vi "PlotFramePositions.vi"() -> ()   [LabVIEW 2012]
panel:
  in  "Frame Size":i16[](array[numeric])
  in  "Coordinates out":dbl[][](array[numeric])
  out "2D Picture":picture
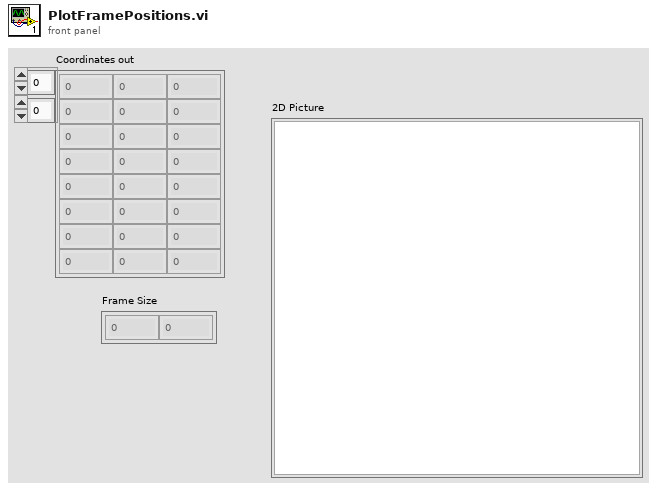
[diagram p1: front panel]
types:
  T1 = cluster{"Width":i16, "Style":enum32{"Solid", "Dash", "Dot", "DashDot", "DashDotDot"}}
  T2 = cluster{"left":i16, "top":i16, "right":i16, "bottom":i16}
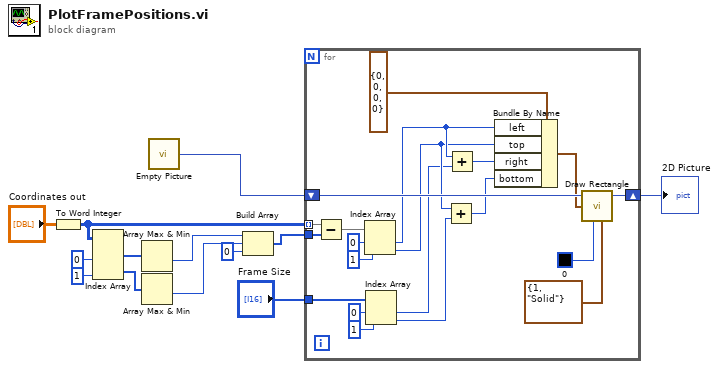
[diagram p0: block diagram]
diagram:
  n1 = To Word Integer(number="Coordinates out") -> (16bit integer=w9:i16[][])
  n2 = Index Array(array=w9, index (col) #1=0 ("disabled index (col)"), index (col) #2=1 ("index (col)")) -> (element #1=w6:i16[], element #2=w5:i16[])  [unwired: 2 in]
  n3 = Array Max & Min(array=w6) -> (min value=w3:i16)  [unwired: 3 out]
  n4 = Array Max & Min(array=w5) -> (min value=w2:i16)  [unwired: 3 out]
  n5 = call "Empty Picture"() -> ("empty picture"=w13:picture)
  n6 = Build Array(w3, w2, i16 0 ("element")) -> (w4:i16[])
  n7 = for {
    tunnel: w9 -> [w17] mode=indexing
    shift-right: [w30] -> w12
    shift-left: w13 -> [w31]
    tunnel: "Frame Size" -> [w20]
    tunnel: w4 -> [w14]
    n8 = Subtract(x=w17, y=w14) -> (x-y=w15:i16[])
    n9 = Index Array(array=w15, index #1=0 ("index"), index #2=1 ("index")) -> (element #1=w25:i16, element #2=w23:i16)
    n10 = Index Array(array=w20, index #1=0 ("index"), index #2=1 ("index")) -> (element #1=w19:i16, element #2=w18:i16)
    n11 = Add(x=w23, y=w18) -> (x+y=w24:i16)
    n12 = Add(x=w25, y=w19) -> (x+y=w26:i16)
    n13 = Bundle By Name(cluster=T2 {"left"=0, "top"=0, "right"=0, "bottom"=0} ("rect"), "left"=w25, "top"=w23, "right"=w26, "bottom"=w24) -> (w28:T2)
    n14 = call <vilib>:"Draw Rectangle.vi"("picture"=w31, "rect"=w28, "color(black)"=u32 0, "pen"=T1 {"Width"=1, "Style"=enum."Solid"}) -> ("new picture"=w30:picture)  [unwired: 5 in]
  }
  "2D Picture" <- w12
